vi "zad7.vi"() -> ()   [LabVIEW 2018]
panel:
  in  "file path":path
  out "Time Signal":waveform(dbl)[](graph)
  in  "?":bool
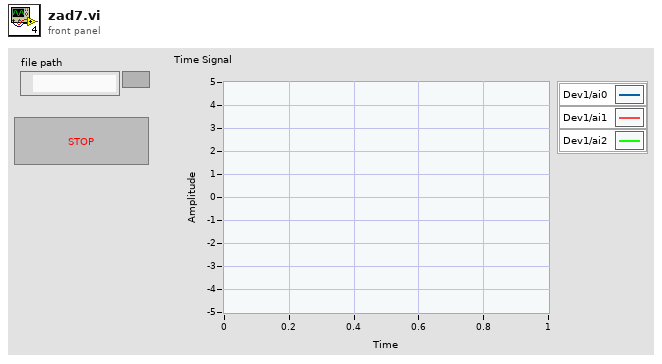
[diagram p1: front panel]
types:
  T1 = enum16{"open", "open or create", "create or replace", "create", "open (read-only)"}
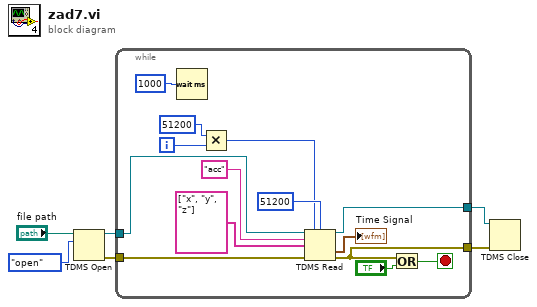
[diagram p0: block diagram]
diagram:
  n1 = TDMS Open(10:T1."open" ("operation (0:open)"), 11:"file path") -> (0:w2:errorcluster, 3:w4:refnum<k34>)  [unwired: 5 in]
  n2 = while {
    tunnel: w4 -> [w20]
    tunnel: [w19] -> w3
    tunnel: w2 -> [w18]
    tunnel: [w13] -> w1
    i -> [w9]
    stop <- w14 stop-if-true
    n3 = Wait (ms)(milliseconds to wait=u32 1000) -> ()  [unwired: 1 out]
    n4 = Multiply(x=i64 51200 ("offset (0)"), y=w9) -> (x*y=w8:i64)
    n5 = TDMS Read(0:w20, 1:w8, 2:i64 51200 ("count (-1: all)"), 5:"acc" ("group name in"), 7:string[] ["x", "y", "z"] ("channel name(s) in"), 11:w18) -> (4:w19:refnum<k34>, 10:→"Time Signal":waveform(dbl)[], 15:w13:errorcluster)  [unwired: 2 in, 3 out]
    n6 = Or(x=w13, y="?") -> (x .or. y?=w14:bool)
  }
  n7 = TDMS Close(8:w1, 11:w3) -> ()  [unwired: 2 out]
